vi "Setup UI.vi"(8 "error in (no error)":errorcluster, 10 "Set UI to input? (F)":bool, 11 "Translation Stage Coarse In":refnum<class "Translation Stage Coarse.lvclass">) -> (0 "error out":errorcluster, 3 "Translation Stage Coarse Out":refnum<class "Translation Stage Coarse.lvclass">)   [LabVIEW 2017, in "Translation Stage Coarse.lvclass"]
uses:
  Translation Stage Coarse.lvclass
  Global/GPIB Numbers.vi
panel:
  in  "Calibrate Zero":bool
  in  "Go to first point":bool
  # "PURE VIRTUAL\nMETHOD CALLED!"
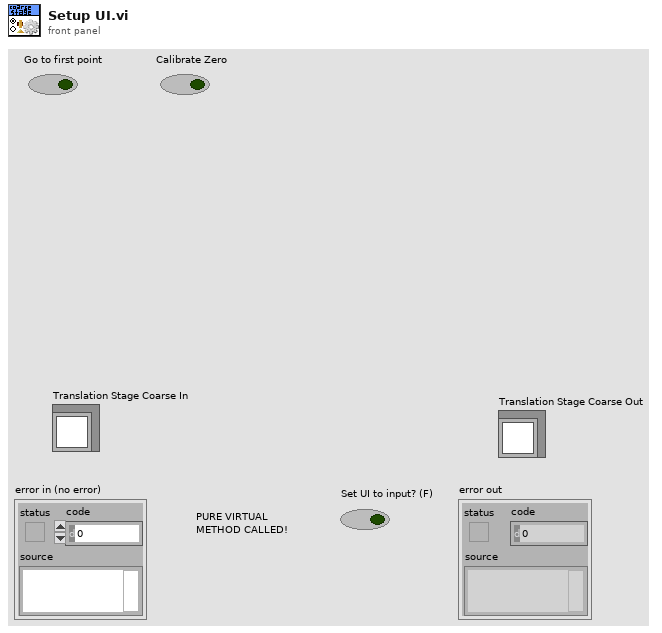
[diagram p1: front panel]
types:
  T1 = typedef "GPIB Type Def.ctl" = cluster{"Name":string, "bus":dbl, "GPIB":dbl, "GPIB as string":string, "byte":i32, "VISA Resource Name":refnum<visa-resource-name>}
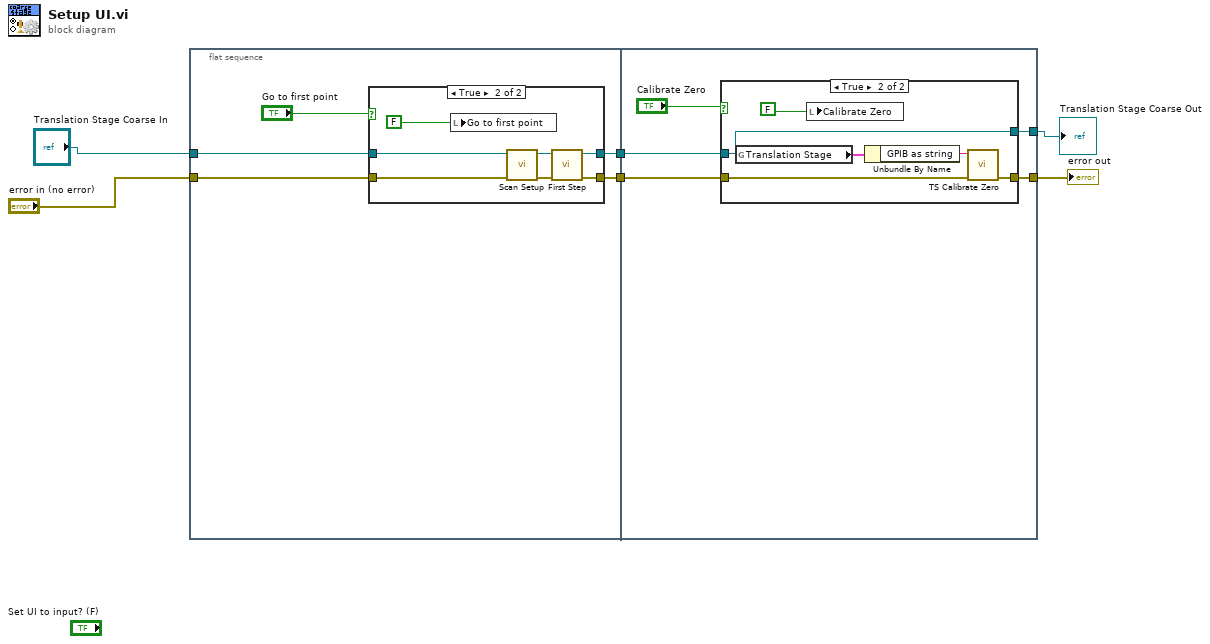
[diagram p0: block diagram]
diagram:
  n1 = flat-sequence {
    tunnel: [w11] -> w6
    tunnel: [w10] -> w5
    tunnel: "Translation Stage Coarse In" -> [w8]
    tunnel: "error in (no error)" -> [w7]
    tunnel: [w24] -> w1
    tunnel: [w22] -> w2
    tunnel: w6 -> [w23]
    tunnel: w5 -> [w25]
    frame #0 {
      n2 = case shown="True" "Go to first point" {
        tunnel: [w12 w17] -> w11
        tunnel: [w13 w16] -> w10
        tunnel: w8 -> [w13 w15]
        tunnel: w7 -> [w12 w14]
        frame False {
        }
        frame True {
          n3 = local write "Go to first point"(FALSE ("Send conds for first point to PG")) -> ()
          n4 = call-dynamic "Scan Setup.vi"("error in (no error)"=w14, "Translation Stage Coarse in"=w15) -> ("error out"=w18:errorcluster, "Translation Stage Coarse out"=w19:refnum<class "Translation Stage Coarse.lvclass">)  [unwired: 8 out]
          n5 = call-dynamic "First Step.vi"("error in (no error)"=w18, "Translation Stage Coarse.lvclass in"=w19) -> ("error out"=w17:errorcluster, "Translation Stage Coarse.lvclass out"=w16:refnum<class "Translation Stage Coarse.lvclass">)  [unwired: 8 out]
        }
      }
    }
    frame #1 {
      n6 = case shown="True" "Calibrate Zero" {
        tunnel: [w27 w29] -> w22
        tunnel: [w26 w30] -> w24
        tunnel: w25 -> [w26 w30]
        tunnel: w23 -> [w27 w31]
        frame False {
        }
        frame True {
          n7 = global read "GPIB Numbers.vi" "Translation Stage"() -> (w33:T1)
          n8 = local write "Calibrate Zero"(FALSE ("Send conds for first point to PG")) -> ()
          n9 = Unbundle By Name(w33) -> ("GPIB as string"=w32:string)
          n10 = call "TS Calibrate Zero.vi"("error out"=w31, "GPIB as string"=w32) -> ("error out 2"=w29:errorcluster)  [unwired: 9 out]
        }
      }
    }
  }
  "error out" <- w2
  "Translation Stage Coarse Out" <- w1
